vi "例4-25.vi"() -> ()   [LabVIEW 2019]
panel:
  out "记录时间":string
  out "记录波形":dbl[](graph)
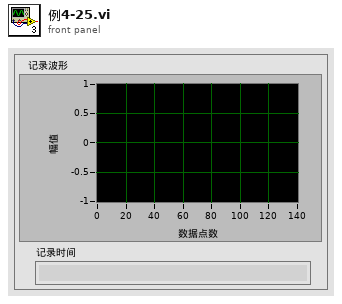
[diagram p1: front panel]
types:
  T1 = enum16{"open", "replace", "create", "open or create", "replace or create", "replace or create with confirmation"}
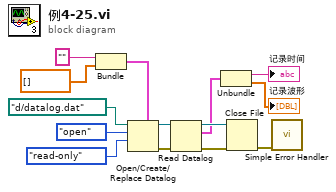
[diagram p0: block diagram]
diagram:
  n1 = Bundle("", dbl[] []) -> (w5:cluster{string, dbl[]})  [unwired: 1 in]
  n2 = Open/Create/Replace Datalog(5:w5, 9:enum16{"read/write", "read-only", "write-only"}."read-only" ("权限(0:read/write)"), 10:T1."open" ("操作(0:open)"), 11:path "d:/datalog.dat" ("数据记录路径（使用对话框）")) -> (0:w10:errorcluster, 3:w4:refnum<k1>)  [unwired: 2 in, 1 out]
  n3 = Read Datalog(4:w10, 7:w4) -> (0:w8:errorcluster, 2:w3:cluster{string, dbl[]}, 3:w9:refnum<k1>)  [unwired: 1 in]
  n4 = Unbundle(w3) -> (→"记录时间":string, →"记录波形":dbl[])
  n5 = Close File(refnum=w9, error in=w8) -> (error out=w14:errorcluster)  [unwired: 1 out]
  n6 = call <vilib>:"Simple Error Handler.vi"("error in (no error)"=w14) -> ()  [unwired: 4 in, 5 out]
